vi "Update PMG.vi"(8 "error in (no error)":errorcluster, 11 "Pump_1AI_1DO_2DI in":refnum<class "PM_Group.lvclass">) -> (0 "error out":errorcluster, 3 "Pump_1AI_1DO_2DI out":refnum<class "PM_Group.lvclass">)   [LabVIEW 2019, in "PM_Group.lvclass"]
uses:
  PM_Group.lvclass
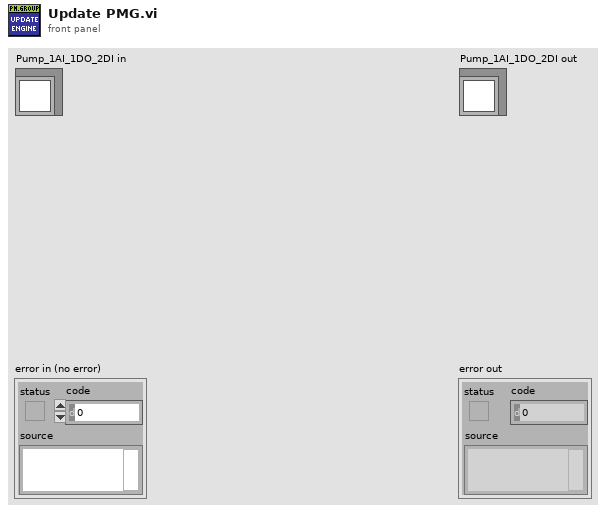
[diagram p1: front panel]
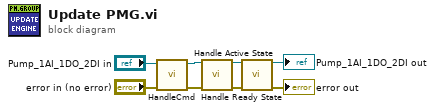
[diagram p0: block diagram]
diagram:
  n1 = call "HandleCmd.vi"("error in (no error)"="error in (no error)", "PM_Group in"="Pump_1AI_1DO_2DI in") -> ("error out"=w2:errorcluster, "PM_Group out"=w3:refnum<class "PM_Group.lvclass">)  [unwired: 8 in]
  n2 = call "Handle Ready State.vi"("reference in"=w3, "error in (no error)"=w2) -> ("reference out"=w8:refnum<class "PM_Group.lvclass">, "error out"=w7:errorcluster)  [unwired: 12 in]
  n3 = call "Handle Active State.vi"("reference in"=w8, "error in (no error)"=w7) -> ("reference out"=→"Pump_1AI_1DO_2DI out":refnum<class "PM_Group.lvclass">, "error out"=→"error out":errorcluster)  [unwired: 12 in]
